vi "Check Refnum Type.vi"(8 "error in (no error)":errorcluster, 11 "Button in":refnum<class "Button.lvclass">) -> (0 "error out":errorcluster, 3 "Button out":refnum<class "Button.lvclass">)   [LabVIEW 2020, in "Button.lvlib" / "Button.lvclass"]
uses:
  Button.lvclass
  Button.lvclass/Button.ctl
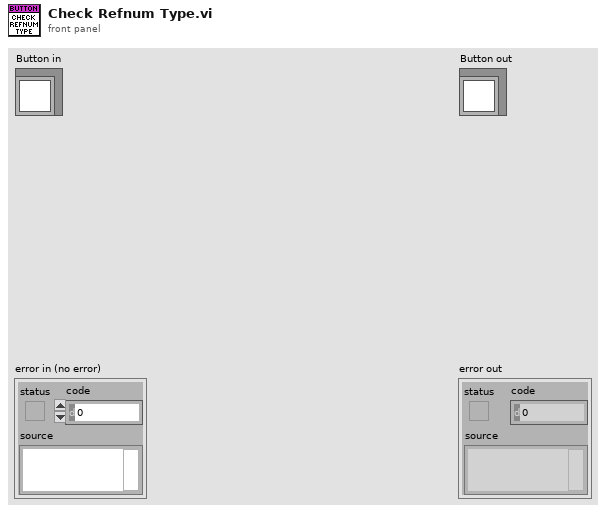
[diagram p1: front panel]
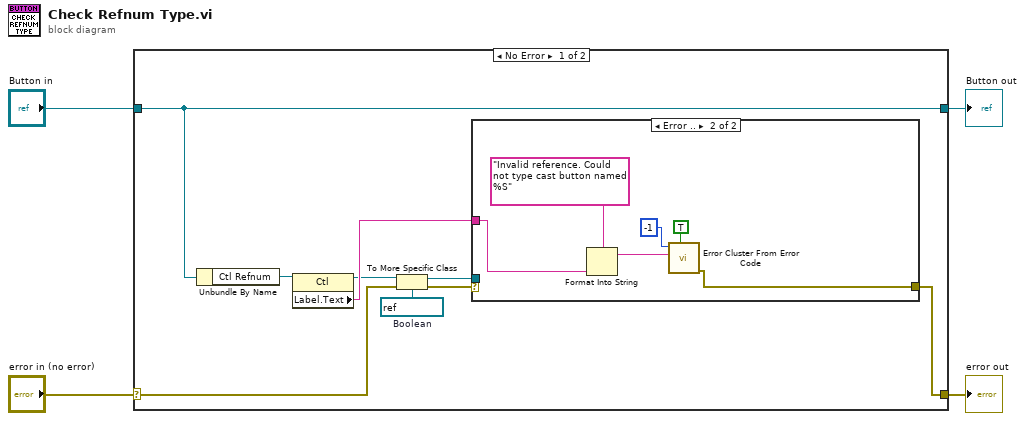
[diagram p0: block diagram]
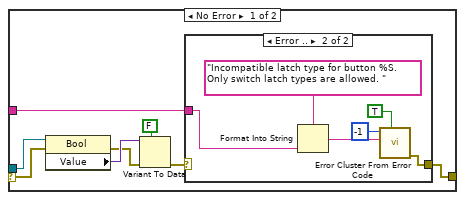
[diagram p2: hidden frame]
diagram:
  n1 = case shown="No Error" "error in (no error)" {
    selector: "error in (no error)" -> [w12 w36]
    tunnel: [w5 w36] -> w3
    tunnel: [w13 w35] -> w1
    tunnel: "Button in" -> [w13 w35]
    frame No Error {
      w10 = refnum<vi> refnum  # Boolean
      n2 = Unbundle By Name(w13) -> ("Ctl Refnum"=w8:refnum<vi>)
      n3 = property class="Ctl"(reference=w8) -> (reference out=w7:refnum<vi>, "Label.Text"=w9:string)  [unwired: 1 in, 1 out]
      n4 = To More Specific Class(target class=w10, reference=w7, error in=w12) -> (specific class reference=w6:refnum<vi>, error out=w11:errorcluster)
      n5 = case shown="Error .." w11 {
        selector: w11 -> [w17 _]
        tunnel: w6 -> [w21 _]
        tunnel: [w15 w31] -> w5
        tunnel: w9 -> [w14 w29]
        frame No Error {
          n6 = property class="Bool"(reference=w21, error in=w17) -> (error out=w18:errorcluster, "Value"=w20:variant)  [unwired: 1 out]
          n7 = Variant To Data(error in=w18, type=FALSE, Variant=w20) -> (error out=w16:errorcluster)  [unwired: 1 out]
          n8 = case shown="Error .." w16 {
            selector: w16 -> [w22 _]
            tunnel: [w22 w23] -> w15
            tunnel: w14 -> [_ w24]
            frame No Error {
            }
            frame Error {
              n9 = Format Into String(format string="Incompatible latch type for button %S. Only switch latch types are allowed. " ("error message (\"\")"), w24) -> (resulting string=w28:string)  [unwired: 2 in, 1 out]
              n10 = call <vilib>:"Error Cluster From Error Code.vi"("show call chain? (False)"=TRUE, "error message (\"\")"=w28, "error code (0)"=-1) -> ("error out"=w23:errorcluster)  [unwired: 6 in]
            }
          }
        }
        frame Error {
          n11 = Format Into String(format string="Invalid reference. Could not type cast button named %S" ("error message (\"\")"), w29) -> (resulting string=w30:string)  [unwired: 2 in, 1 out]
          n12 = call <vilib>:"Error Cluster From Error Code.vi"("show call chain? (False)"=TRUE, "error message (\"\")"=w30, "error code (0)"=-1) -> ("error out"=w31:errorcluster)  [unwired: 6 in]
        }
      }
    }
    frame Error {
    }
  }
  "error out" <- w3
  "Button out" <- w1
